vi "OE2011&OE2021_Query Signal Data.vi"(0 "VISA resource name":refnum<visa-resource-name>, 5 "Connection ID in":refnum<k5>, 7 "Remote Mode":u16(ring) items=["USB", "RS232", "GPIB", "Ethernet"], 9 "Query Type":u16(ring)=3 items=["X-Demod1", "Y-Demod1", "R-Demod1", "Theta-Demod1", "X-Demod2", "Y-Demod2", "R-Demod2", "Theta-Demod2", "X-Demod3", "Y-Demod3", "R-Demod3", "Theta-Demod3", "X-Demod4", "Y-Demod4", "R-Demod4", "Theta-Demod4", "X-Demod5", "Y-Demod5", "R-Demod5", "Theta-Demod5", "X-Demod6", "Y-Demod6", "R-Demod6", "Theta-Demod6", "X-Demod7", "Y-Demod7", "R-Demod7", "Theta-Demod7", "X-Demod8", "Y-Demod8", "R-Demod8", "Theta-Demod8", "Xnoisd-Demod1", "Ynoisd-Demod1", "Xnoisd-Demod5", "Ynoisd-Demod5", "Frequency-OSC1", "Frequency-OSC2", "AUXIN1", "AUXIN2", "AUXIN3", "AUXIN4", "Timestamps"], 11 "Error in (no error)":errorcluster caption="error out（no error）") -> (4 "VISA resource  out":refnum<visa-resource-name>, 6 "Connection ID out":refnum<k5>, 8 "Read Buffer":string, 10 "Output String":string, 15 "Error out":errorcluster caption="error out")   [LabVIEW 2011]
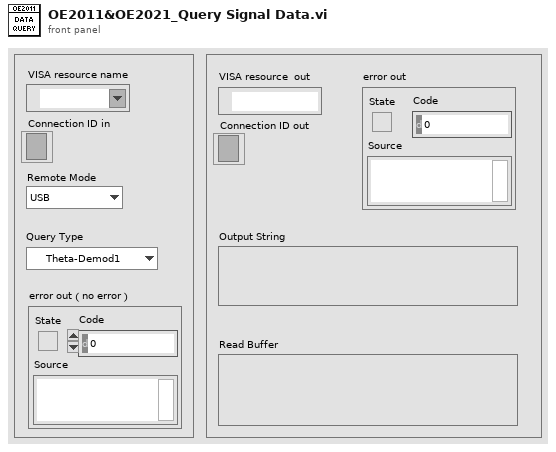
[diagram p1: front panel]
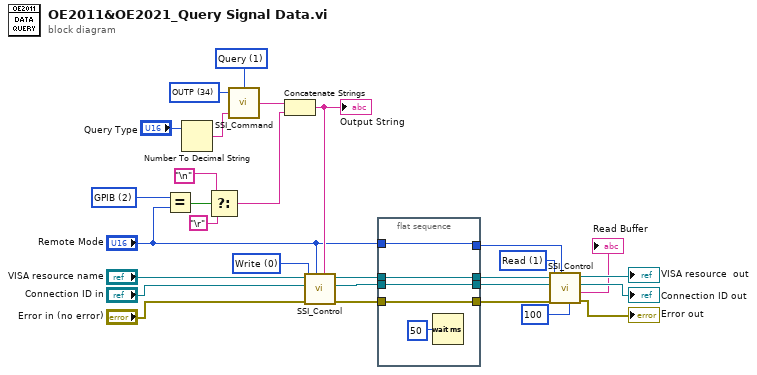
[diagram p0: block diagram]
diagram:
  w11 = u16 2 items=["USB", "RS232", "GPIB", "Ethernet"] ("Remote Mode")
  w21 = u16 34 items=["ISRC", "IGND", "ICPL", "ILIN", "PHAS", "FMOD", "RSLP", "FREQ", "SWPT", "SLLM", "SULM", "SSLL", "SSLG", "STLM", "SWRM", "IRNG", "SENS", "RMOD", "OFLT", "OFSL", "SYNC", "DMOD", "HARM", "DARB", "SWVT", "SLVL", "SVLL", "SVUL", "SVSL", "SVSG", "SVTM", "SVRM", "RALL", "SNAP", "OUTP", "OAUX", "COUT", "CAUX", "COFP", "CEXP", "FPOP", "OEXP", "*IDN", "*RST", "OVLD", "INOV", "GNOV", "*PLL", "SSET", "RSET", "AGAN", "APHS", "ARSV", "ASCL", "EQCD", "EQCS", "SPED", "SRAT", "SLEN", "SSLE", "STRG", "SPRM", "STRD", "PAUS", "RSET", "SPTS", "TRCA", "TEMP", "RSTU", "INHZ", "DEQU", "SADD", "ARNG", "CSPE", "ISRCD", "IGNDD", "ICPLD", "ILIND", "PHASD", "FMODD", "RSLPD", "FREQD", "SWPTD", "SLLMD", "SULMD", "SSLLD", "SSLGD", "STLMD", "SWRMD", "SENSD", "RMODD", "OFLTD", "OFSLD", "SYNCD", "HARMD", "EQCDD", "EQCSD", "SNAPD", "OUTPD", "SWVTD", "SLVLD", "SVLLD", "SVULD", "SVSLD", "SVSGD", "SVTMD", "SVRMD", "SVDCD", "ARSVD", "AGAND", "APHSD", "ASCLD", "FPOPD", "CAUXD", "OEXPD", "SPEDD", "SRATD", "SLEND", "SSLED", "STRGD", "SPRMD", "STRDD", "PAUSD", "RESTD", "SPTSD", "TRCAD", "*IDND", "*RSTD", "INOVD", "GNOVD", "*PLLD", "SSETD", "RSETD", "RALLD"] ("Command Type")
  w19 = u16 1 items=["Set", "Query"] ("Opera")
  w24 = u16 1 items=["Write", "Read"] ("Control")
  w29 = u16 0 items=["Write", "Read"] ("Control")
  n1 = Equal?(x=w11, y="Remote Mode") -> (x = y?=w6:bool)
  n2 = Number To Decimal String(number="Query Type") -> (decimal integer string=w14:string)  [unwired: 1 in]
  n3 = Select(t="\n", s=w6, f="\r") -> (s? t:f=w9:string)
  n4 = call "SSI_Command.vi"("Opera"=w19, "Paramter"=w14, "Command Type"=w21) -> ("Output string"=w20:string)  [unwired: 1 in]
  n5 = Concatenate Strings(w20, w9) -> (w22:string)
  "Output String" <- w22
  n6 = call "SSI_Control.vi"("Write Buffer"=w22, "Remote Mode"="Remote Mode", "Error in (no error)"="Error in (no error)", "Control"=w29, "Connection ID in"="Connection ID in", "VISA resource name"="VISA resource name") -> ("Error out"=w27:errorcluster, "Connection ID out"=w2:refnum<k5>, "VISA resource  out"=w28:refnum<visa-resource-name>)  [unwired: 2 in, 1 out]
  n7 = flat-sequence {
    tunnel: w28 -> [w34]
    tunnel: w27 -> [w33]
    tunnel: [w34] -> w26
    tunnel: [w33] -> w25
    tunnel: [w31] -> w23
    tunnel: "Remote Mode" -> [w31]
    tunnel: [w30] -> w3
    tunnel: w2 -> [w30]
    frame #0 {
      n8 = Wait (ms)(milliseconds to wait=u32 50 ("等待时间（毫秒）")) -> ()  [unwired: 1 out]
    }
  }
  n9 = call "SSI_Control.vi"("Tineout"=100, "Remote Mode"=w23, "Error in (no error)"=w25, "Control"=w24, "Connection ID in"=w3, "VISA resource name"=w26) -> ("Error out"=→"Error out":errorcluster, "Read Buffer"=→"Read Buffer":string, "Connection ID out"=→"Connection ID out":refnum<k5>, "VISA resource  out"=→"VISA resource  out":refnum<visa-resource-name>)  [unwired: 2 in]
